vi "Get All Other E2E Nodes.vi"(8 "error in (no error)":errorcluster, 11 "E2E editor node in":refnum<data-value>) -> (0 "error out":errorcluster, 2 "Other E2E editor nodes":refnum<data-value>[](array[refnum]), 3 "E2E editor node out":refnum<data-value>)   [LabVIEW 2015, in "E2E Tag Exchange editor node.lvclass"]
uses:
  E2E Tag Exchange editor node.lvclass
  <vilib>/NI/Configuration Framework/Node/NISE_CEF_Node.lvclass
  Node LUT/Command.ctl
  Node LUT/Node LUT.lvlib
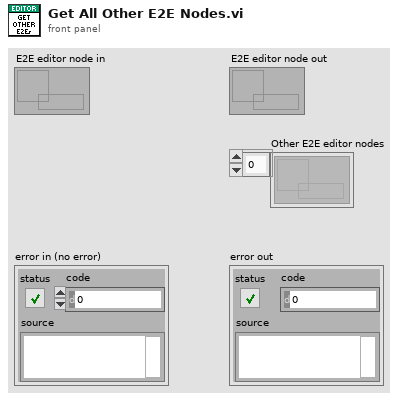
[diagram p1: front panel]
types:
  T1 = typedef "Node LUT.lvlib/Command.ctl" = enum16{"Initialize", "Add Node", "Remove Node", "Node Ref from UID", "List Nodes"}
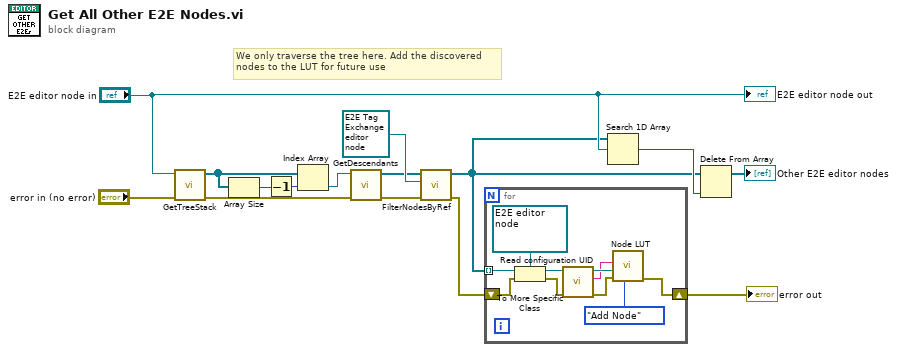
[diagram p0: block diagram]
diagram:
  # "We only traverse the tree here. Add the discovered\nnodes to the LUT for future use"
  n1 = call <vilib>:"GetTreeStack.vi"("error in"="error in (no error)", "node in"="E2E editor node in") -> ("error out"=w8:errorcluster, "parents"=w4:refnum<data-value>[])  [unwired: 8 in]
  n2 = Array Size(array=w4) -> (size(s)=w5:i32)
  n3 = Decrement(x=w5) -> (x-1=w6:i32)
  n4 = Index Array(array=w4, index=w6) -> (element=w7:refnum<data-value>)
  n5 = call <vilib>:"GetDescendants.vi"("error in"=w8, "node in"=w7) -> ("error out"=w11:errorcluster, "descendants"=w9:refnum<data-value>[])  [unwired: 8 in]
  n6 = call <vilib>:"FilterNodesByRef.vi"("error in"=w11, "NISE_CEF_Node"=refnum<class "E2E Tag Exchange editor node.lvclass"> refnum ("E2E editor node"), "nodes"=w9) -> ("error out"=w2:errorcluster, "filtered nodes"=w3:refnum<data-value>[])  [unwired: 7 in]
  n7 = for {
    tunnel: w3 -> [w24] mode=indexing
    shift-right: [w19] -> w1
    shift-left: w2 -> [w18]
    n8 = To More Specific Class(target class=refnum<data-value> refnum, reference=w24, error in=w18) -> (specific class reference=w23:refnum<data-value>, error out=w17:errorcluster)
    n9 = call "Read configuration UID.vi"("error in (no error)"=w17, "E2E editor node in"=w23) -> ("error out"=w21:errorcluster, "Module UID"=w20:string, "E2E editor node out"=w25:refnum<data-value>)  [unwired: 7 in]
    n10 = call "Node LUT.vi"("Command"=Command."Add Node", "error in"=w21, "node ref"=w25, "UID"=w20) -> ("error out"=w19:errorcluster)  [unwired: 4 in, 3 out]
  }
  "error out" <- w1
  n11 = Search 1D Array(1D array=w3, element="E2E editor node in") -> (index of element=w14:i32)  [unwired: 1 in]
  n12 = Delete From Array(array=w3, index=w14) -> (array with subset deleted=→"Other E2E editor nodes":refnum<data-value>[])  [unwired: 1 in, 1 out]
  "E2E editor node out" <- "E2E editor node in"
